vi "ReadInHeightSurvey.vi"(1 "VP.TTHeightCorrs In":T1={"Use Height Corrections"=TRUE, "TT.Azimuths"=[], "Z.HeightCorrs"=[], "Corrections from File"=TRUE, "Height Survey Filepaths"=[]}) -> (0 "VP.TTHeightCorrs Out":T1={"Use Height Corrections"=TRUE, "TT.Azimuths"=[], "Z.HeightCorrs"=[], "Corrections from File"=TRUE, "Height Survey Filepaths"=[]})   [LabVIEW 2015]
uses:
  MultirunBuilderSubVIs/CorrectionsCluster.ctl
  <vilib>/Utility/file.llb/Read Delimited Spreadsheet (DBL).vi
panel:
  out "Height Survey File Data":dbl[][](array[numeric])
  # "<Column 1> TurnTable Azimuth [deg]\n<Column 2> X [mm]\n<Column 3> Y [mm]\n<Column 4> Z [mm]\n<Column 5> Zsensor [mm]"
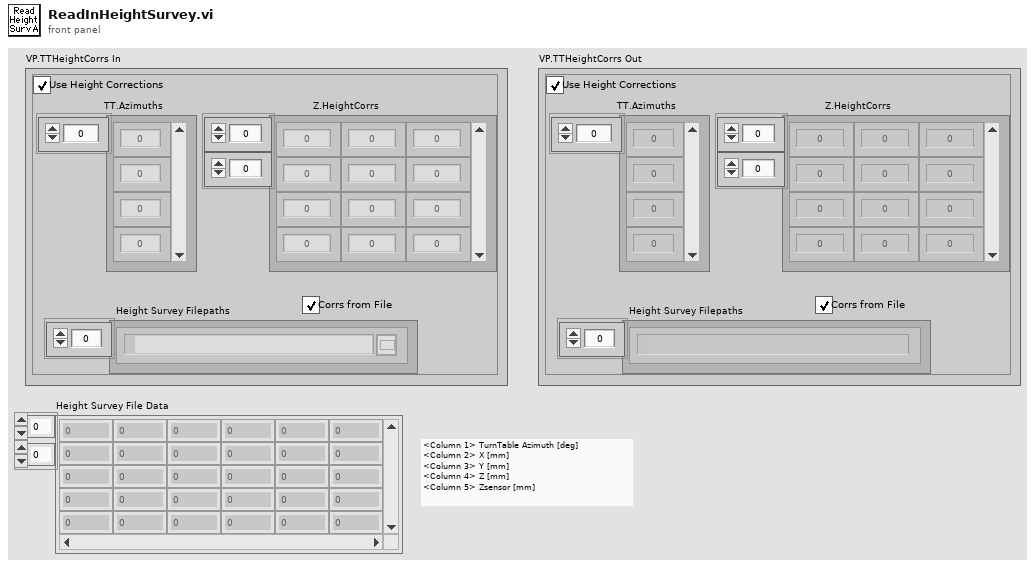
[diagram p1: front panel]
types:
  T1 = typedef "CorrectionsCluster.ctl" = cluster{"Use Height Corrections":bool, "TT.Azimuths":dbl[], "Z.HeightCorrs":dbl[][], "Corrections from File":bool, "Height Survey Filepaths":path[]}
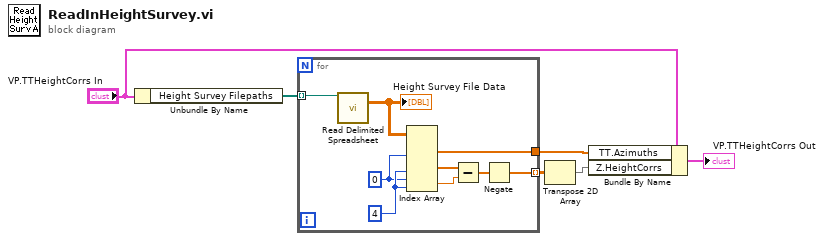
[diagram p0: block diagram]
diagram:
  n1 = Unbundle By Name("VP.TTHeightCorrs In") -> ("Height Survey Filepaths"=w3:path[])
  n2 = for {
    tunnel: w3 -> [w15] mode=indexing
    tunnel: [w13] -> w6
    tunnel: [w8] -> w4 mode=indexing
    w12 = 4 ("index (col)")
    w7 = 0 ("disabled index (col)")
    n3 = call-poly <vilib>:"Read Delimited Spreadsheet.vi"("file path (dialog if empty)"=w15) -> ("all rows"=w14:dbl[][])  [unwired: 9 in, 5 out]
    "Height Survey File Data" <- w14
    n4 = Index Array(array=w14, index (col) #1=w7, index (col) #2=w12, index (row) #3=w7, index (col) #3=w12) -> (element #1=w13:dbl[], element #2=w11:dbl[], element #3=w10:dbl)  [unwired: 2 in]
    n5 = Subtract(x=w11, y=w10) -> (x-y=w9:dbl[])
    n6 = Negate(x=w9) -> (-x=w8:dbl[])
  }
  n7 = Transpose 2D Array(2D array=w4) -> (transposed array=w5:dbl[][])
  n8 = Bundle By Name(cluster="VP.TTHeightCorrs In", "TT.Azimuths"=w6, "Z.HeightCorrs"=w5) -> (→"VP.TTHeightCorrs Out":T1)
